vi "LabVIEW Datatype to Measurement Datatype.vi"(1 "LabVIEW type":T2) -> (0 "Measurement DataType":T1)   [LabVIEW 2020, in "LoadRegulation.lvlib" / "MeasurementService_Template.lvclass"]
uses:
  MeasurementService_Template.lvclass
  <vilib>/Utility/Data Type/Type Definitions/Data Type.ctl
  Measurement DataType.ctl
  <vilib>/Utility/Data Type/NI_Data Type.lvlib
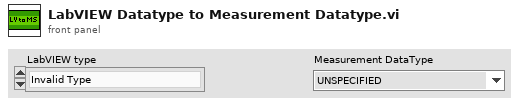
[diagram p1: front panel]
types:
  T1 = typedef "LoadRegulation.lvlib/MeasurementService_Template.lvclass/Measurement DataType.ctl" = enum16{"UNSPECIFIED", "BOOL", "DOUBLE", "FLOAT", "INT32", "INT64", "STRING", "UINT32", "UINT64"}
  T2 = typedef "NI_Data Type.lvlib/Data Type.ctl" = enum8{"Invalid Type", "Void", "I8", "I16", "I32", "I64", "U8", "U16", "U32", "U64", "Single Float", "Double Float", "Extended Float", "Single Complex", "Double Complex", "Extended Complex", "Enum U8", "Enum U16", "Enum U32", "Enum U64", "Single Float With Unit", "Double Float With Unit", "Extended Float With Unit", "Single Complex with Unit", "Double Complex with Unit", "Extended Complex with Unit", "Boolean", "String", "Path", "Picture", "Tag", "Array", "Cluster", "Variant", "LV Variant", "Waveform", "Timestamp", "Digital Waveform", "Digital Data", "ExpressData", "Refnum", "External Data", "VI", "Poly VI", "LabVIEW Class Instance", "Fixed Point", "Set Collection", "Map Collection"}
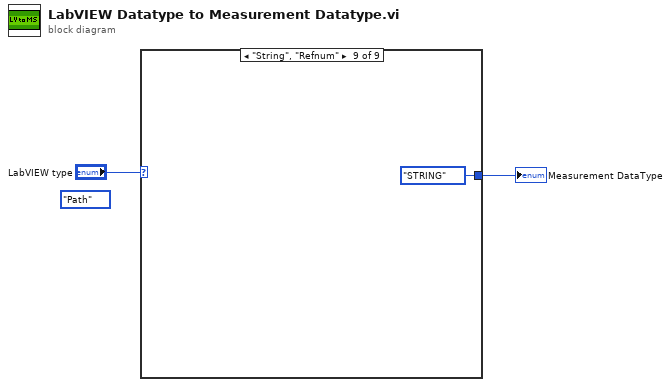
[diagram p0: block diagram]
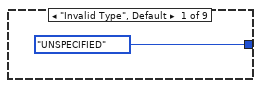
[diagram p2: hidden frame]
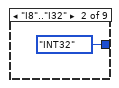
[diagram p3: hidden frame]
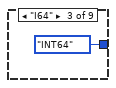
[diagram p4: hidden frame]
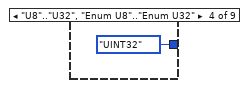
[diagram p5: hidden frame]
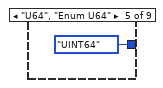
[diagram p6: hidden frame]
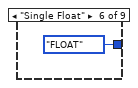
[diagram p7: hidden frame]
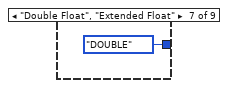
[diagram p8: hidden frame]
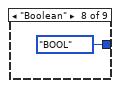
[diagram p9: hidden frame]
diagram:
  (unwired) Data_Type."Path" ("LabVIEW type")
  n1 = case shown="\"String\", \"Refnum\"" "LabVIEW type" {
    tunnel: [Measurement_DataType."UNSPECIFIED" ("Measurement DataType") Measurement_DataType."INT32" ("Measurement DataType") Measurement_DataType."INT64" ("Measurement DataType") Measurement_DataType."UINT32" ("Measurement DataType") Measurement_DataType."UINT64" ("Measurement DataType") Measurement_DataType."FLOAT" ("Measurement DataType") Measurement_DataType."DOUBLE" ("Measurement DataType") Measurement_DataType."BOOL" ("Measurement DataType") Measurement_DataType."STRING" ("Measurement DataType")] -> w1
    frame "Invalid Type", Default {
    }
    frame "I8".."I32" {
    }
    frame "I64" {
    }
    frame "U8".."U32", "Enum U8".."Enum U32" {
    }
    frame "U64", "Enum U64" {
    }
    frame "Single Float" {
    }
    frame "Double Float", "Extended Float" {
    }
    frame "Boolean" {
    }
    frame "String", "Refnum" {
    }
  }
  "Measurement DataType" <- w1
